vi "gu_rotate_string.vi"(8 "error in":errorcluster, 11 "Encoded String in":T1) -> (0 "error out":errorcluster, 3 "Encoded String out":string)   [LabVIEW 2020, in "G-Unicode.lvlib"]
uses:
  G-Unicode.lvlib
  Types/Encoded UTF-8 String.ctl
  lib/g_unicode_32.dll
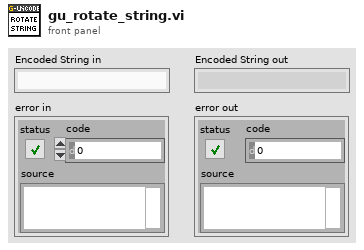
[diagram p1: front panel]
types:
  T1 = typedef "G-Unicode.lvlib/Encoded UTF-8 String.ctl" = string
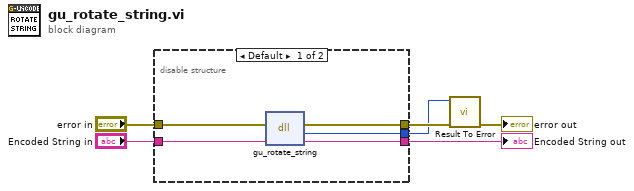
[diagram p0: block diagram]
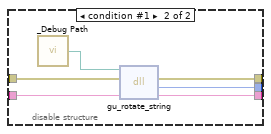
[diagram p2: hidden frame]
diagram:
  n1 = disable-structure shown="Default" {
    disable-tunnel: "Encoded String in" -> [w11 w17]
    disable-tunnel: "error in" -> [w10 w16]
    disable-tunnel: [w9 w15] -> w3
    disable-tunnel: [w8 w14] -> w4
    disable-tunnel: [w7 w12] -> w1
    frame condition #0 (active) {
      n2 = dll-call lib="C:/github/dataflowg/g-unicode/src/LabVIEW/G-Unicode/lib/g_unicode_*.*" fn="gu_rotate_string"(error in=w10, "str"=w11) -> (error out=w9:errorcluster, "result"=w7:i32, "str"=w8:string)  [unwired: 2 in, 1 out]
    }
    frame condition #1 {
      n3 = call "_Debug Path.vi"() -> ("Debug Path"=w13:path)
      n4 = dll-call lib="?" fn="gu_rotate_string"(path in=w13, error in=w16, "str"=w17) -> (error out=w15:errorcluster, "result"=w12:i32, "str"=w14:string)  [unwired: 1 in, 1 out]
    }
  }
  "Encoded String out" <- w4
  n5 = call "Result To Error.vi"("error in (no error)"=w3, "Result Code"=w1) -> ("error out"=→"error out":errorcluster)  [unwired: 9 in]
